vi "logtofile.vi"(0 "LogFile":path, 1 "text":string, 5 "error in (no error)":errorcluster) -> (19 "error out":errorcluster)   [LabVIEW 2014]
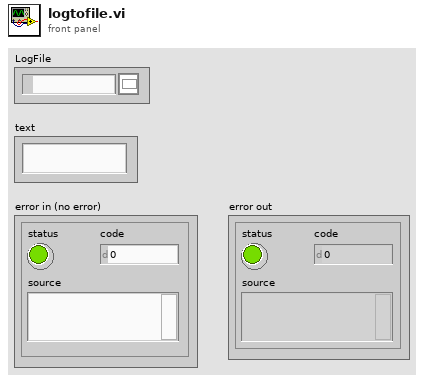
[diagram p1: front panel]
types:
  T1 = enum16{"open", "replace", "create", "open or create", "replace or create", "replace or create with confirmation"}
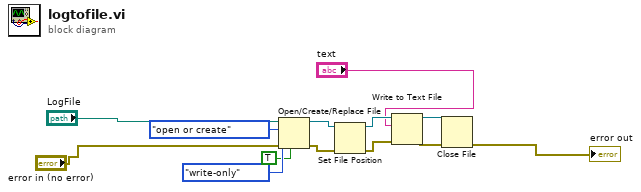
[diagram p0: block diagram]
diagram:
  n1 = Open/Create/Replace File(file path (use dialog)="LogFile", error in="error in (no error)", operation (0:open)=T1."open or create", access (0:read/write)=enum16{"read/write", "read-only", "write-only"}."write-only", disable buffering (F)=TRUE) -> (refnum out=w5:refnum<file>, error out=w8:errorcluster)  [unwired: 1 in, 1 out]
  n2 = Set File Position(refnum=w5, error in=w8) -> (refnum out=w4:refnum<file>, error out=w10:errorcluster)  [unwired: 2 in]
  n3 = Write to Text File(file (use dialog)=w4, text="text", error in=w10) -> (refnum out=w11:refnum<file>, error out=w12:errorcluster)  [unwired: 1 in, 1 out]
  n4 = Close File(refnum=w11, error in=w12) -> (error out=→"error out":errorcluster)  [unwired: 1 out]
